vi "Read Incoming Bytes.vi"(8 "error in (no error)":errorcluster, 9 "timeout (1000 ms)":i32=1000, 10 "bytes to read (100)":i32=100, 11 "WSConnection in":refnum<class "WebsocketsConnection.lvclass">) -> (0 "error out":errorcluster, 1 "timed out":bool, 2 "Bytes":u8[](array[numeric]) format="%08b", 3 "WSConnection":refnum<class "WebsocketsConnection.lvclass">, 4 "connected":bool)   [LabVIEW 2013, in "MQTT_Websockets.lvlib" / "WebsocketsConnection.lvclass"]
uses:
  WebsocketsConnection.lvclass
  WebsocketsConnection.lvclass/WebsocketsConnection.ctl
  <vilib>/MediaMongrels Ltd/WebSockets/WebSockets/WebSocket/WebSocket.lvclass
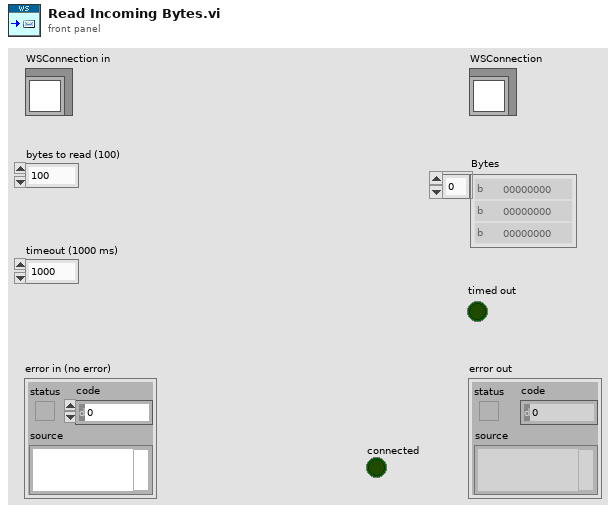
[diagram p1: front panel]
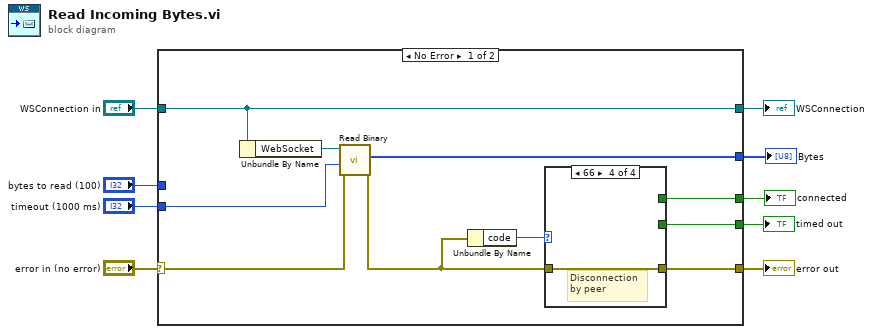
[diagram p0: block diagram]
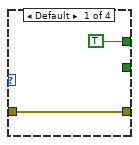
[diagram p2: hidden frame]
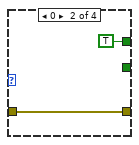
[diagram p3: hidden frame]
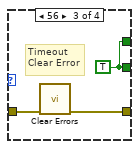
[diagram p4: hidden frame]
diagram:
  n1 = case shown="No Error" "error in (no error)" {
    selector: "error in (no error)" -> [w11 w29]
    tunnel: [w16 w29] -> w8
    tunnel: [w17 w28] -> w6
    tunnel: "WSConnection in" -> [w17 w28]
    tunnel: [w12 _] -> w5
    tunnel: "bytes to read (100)" -> [_ _]
    tunnel: "timeout (1000 ms)" -> [w13 _]
    tunnel: [w18 _] -> w2
    tunnel: [w15 _] -> w1
    frame No Error {
      n2 = Unbundle By Name(w17) -> ("WebSocket"=w14:refnum<class "WebSocket.lvclass">)
      n3 = call-dynamic "Read Binary.vi"("error in (no error)"=w11, "timeout ms (5000)"=w13, "WebSocket in"=w14) -> ("error out"=w10:errorcluster, "Data"=w12:u8[])  [unwired: 6 in, 1 out]
      n4 = Unbundle By Name(w10) -> ("code"=w19:i32)
      n5 = case shown="66" w19 {
        tunnel: [w21 w23 w26 w27] -> w16
        tunnel: w10 -> [w21 w23 w25 w27]
        tunnel: [_ _ w24 _] -> w18
        tunnel: [TRUE TRUE w24 _] -> w15
        frame Default {
        }
        frame 0 {
        }
        frame 56 {
          w24 = TRUE
          # "Timeout\nClear Error"
          n6 = call <vilib>:"Clear Errors.vi"("error in (no error)"=w25) -> ("error out"=w26:errorcluster)  [unwired: 6 in]
        }
        frame 66 {
          # "Disconnection\nby peer"
        }
      }
    }
    frame Error {
    }
  }
  "error out" <- w8
  "WSConnection" <- w6
  "Bytes" <- w5
  "timed out" <- w2
  "connected" <- w1
